vi "EP_SP.vi"(8 "error in":errorcluster, 10 "new_position":i32, 11 "VISA in":refnum<visa-resource-name>) -> (0 "error out":errorcluster, 3 "VISA out":refnum<visa-resource-name>)   [LabVIEW 2019]
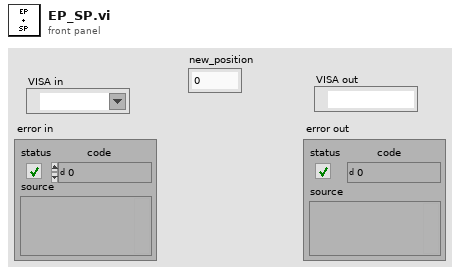
[diagram p1: front panel]
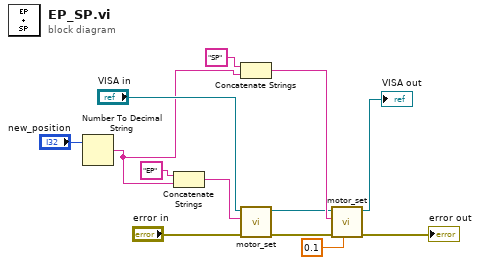
[diagram p0: block diagram]
diagram:
  n1 = Number To Decimal String(number="new_position") -> (decimal integer string=w4:string)  [unwired: 1 in]
  n2 = Concatenate Strings("EP", w4) -> (w13:string)
  n3 = Concatenate Strings("SP", w4) -> (w7:string)
  n4 = call "motor_set.vi"("error in"="error in", "command"=w13, "VISA in"="VISA in") -> ("error out"=w3:errorcluster, "VISA out"=w6:refnum<visa-resource-name>)  [unwired: 7 in]
  n5 = call "motor_set.vi"("delay  (sec)"=0.1, "error in"=w3, "command"=w7, "VISA in"=w6) -> ("error out"=→"error out":errorcluster, "VISA out"=→"VISA out":refnum<visa-resource-name>)  [unwired: 6 in]
